vi "Snap_timestamp.vi"(8 "error in":errorcluster, 10 "Camera":T5, 11 "input cluster":T1={"L16 Linear Actuator"="", "XE 1000 Pump"="", "Camera1"="", "Camera2"="", "Img_Capt"=FALSE, "Actuator"=FALSE, "Pump"=FALSE, "Cam 1"=FALSE, "Cam 2"=FALSE, "Empty_Refill"=FALSE, "Crop"=FALSE, "Light intensity"=100, "Exposure Time"=1000.0, "Sample Name"="Test Sample", "Operator"="MRJ", "Calibration 1"=path "C:/Users/au540322/Desktop/IHS_Project/images/Debris/Debris_0/Debris_0_2019_06_01-23-32-49-686.PNG", "Calibration 2"=path "C:/Users/au540322/Desktop/IHS_Project/images/Debris/Debris_0/Debris_0_2019_06_01-23-32-49-686.PNG", "Framerate"=100, "Timeout Sample"=200, "Collection date"="", "Sample size threshold"=500, "Empty start"=1, "Command"="", "Station"="", "Species Name"="", "Other Notes"="", "Aperture"=enum."Item 0", "Image Process Queue Size"=500, "Image Save Queue Size"=500, "Overload threshold"=500, "Max Framerate"=100, "Rectangle 1"={"Left"=0, "Top"=0, "Right"=0, "Bottom"=0, "Rotation"=0.0}, "Rectangle 2"={"Left"=0, "Top"=0, "Right"=0, "Bottom"=0, "Rotation"=0.0}, "Detection Region %"=0.0, "Detect 1"=path "C:/Users/au540322/Desktop/IHS_Project/images/Debris/Debris_0/Debris_0_2019_06_01-23-32-49-686.PNG", "Detect 2"=path "C:/Users/au540322/Desktop/IHS_Project/images/Debris/Debris_0/Debris_0_2019_06_01-23-32-49-686.PNG", "Max large object threshold"=0, "Open(T)/Close(F)"=FALSE, "Img_Capt Begin"=FALSE, "Dispense Speed"=100, "Flush Size"=100, "Location"="Station", "Latitude"="Station", "Longitude"="Station", "Determiner"="Station", "Sex"="Station", "Camera1_Img"=refnum, "Camera2_Img"=refnum, "Img1_Orig_Disp"=refnum, "Img2_Orig_Disp"=refnum, "Img1_Orig_RGB"=refnum, "Img2_Orig_RGB"=refnum, "Blue_Plane_Extract"=refnum, "Subtracted_Plane"=refnum, "Img1_Binary"=refnum, "Img2_Binary"=refnum, "Crop_Mask"=refnum, "Img1_Save"=refnum, "Img2_Save"=refnum, "Img1_Cali_Full"=refnum, "Img2_Cali_Full"=refnum, "Img1_Cali_Detect"=refnum, "Img2_Cali_Detect"=refnum, "Cam 1 queue"=refnum, "Cam 2 queue"=refnum, "Cam 1 - save queue"=refnum, "Cam 2 - save queue"=refnum, "Overlay_Ring"=0, "SystemVersion"=0, "System Serial"="", "Legacy Cam Attributes"=FALSE} {"SystemVersion" items=["Standard", "XL"]; "Overlay_Ring" items=["Session Data", "Extended Setup", "Buffer", "Camera", "Dispenser", "Stats", "Connections"]; "Flush Size" min=1; "Dispense Speed" min=1; "Rectangle 2"."Rotation" format="%.2f"; "Rectangle 2"."Left" scale=0.0..1024.0; "Rectangle 2"."Right" scale=0.0..1024.0; "Rectangle 1"."Rotation" format="%.2f"; "Rectangle 1"."Left" scale=0.0..1024.0; "Rectangle 1"."Right" scale=0.0..1024.0; "Max Framerate" min=1; "Overload threshold" min=1; "Image Save Queue Size" min=1; "Image Process Queue Size" min=1; "Empty start" min=1; "Sample size threshold" min=1; "Framerate" min=1; "Light intensity" scale=0.0..100.0}) -> (0 "error out":errorcluster)   [LabVIEW 2022 SP3]
uses:
  Camera_ID.ctl
  controls/Data.ctl
  <vilib>/userdefined/High Color/IMAQdx.ctl
  <vilib>/vision/Image Controls.llb/IMAQ Image.ctl
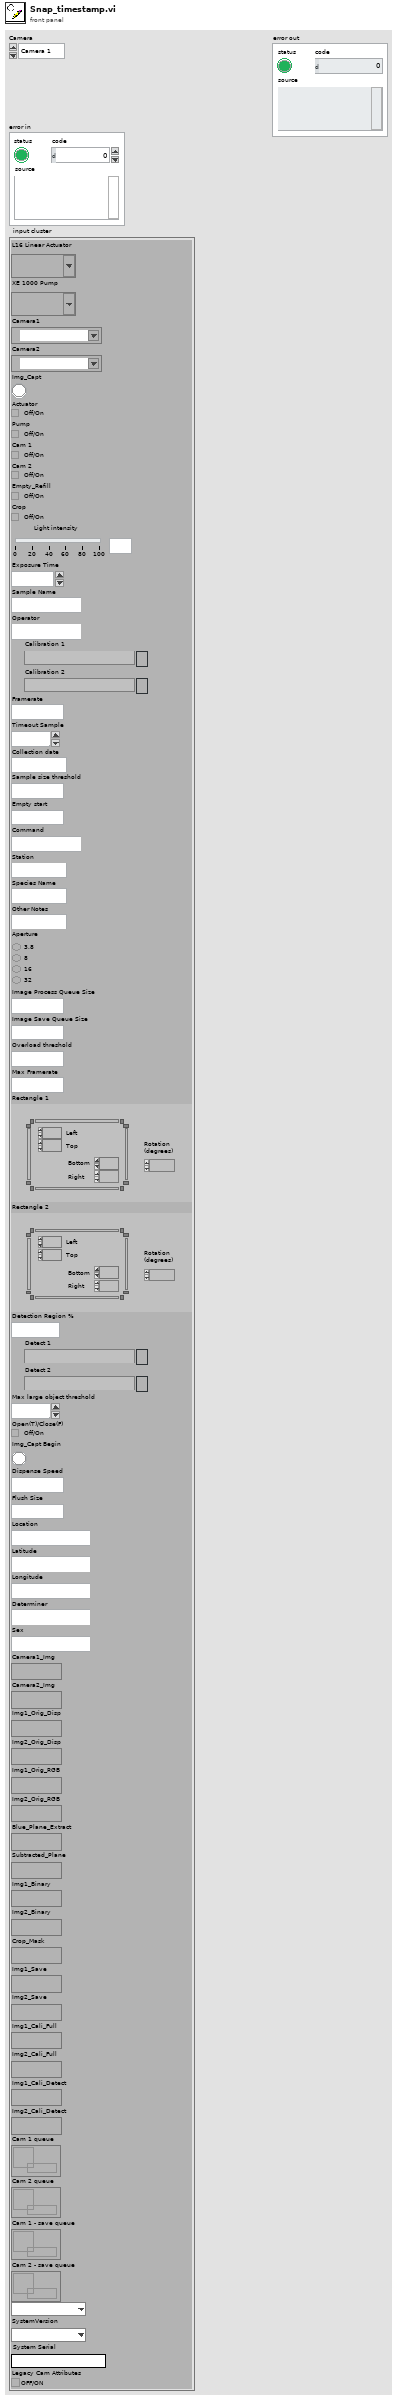
[diagram p1: front panel]
types:
  T1 = typedef "Data.ctl" = cluster{"L16 Linear Actuator":refnum<visa-resource-name>, "XE 1000 Pump":refnum<visa-resource-name>, "Camera1":T2, "Camera2":T2, "Img_Capt":bool, "Actuator":bool, "Pump":bool, "Cam 1":bool, "Cam 2":bool, "Empty_Refill":bool, "Crop":bool, "Light intensity":i32, "Exposure Time":dbl, "Sample Name":string, "Operator":string, "Calibration 1":path, "Calibration 2":path, "Framerate":i32, "Timeout Sample":i32, "Collection date":string, "Sample size threshold":i32, "Empty start":u32, "Command":string, "Station":string, "Species Name":string, "Other Notes":string, "Aperture":enum32{"Item 0", "Item 1", "Item 2", "Item 3"}, "Image Process Queue Size":i32, "Image Save Queue Size":i32, "Overload threshold":i32, "Max Framerate":i32, "Rectangle 1":T3, "Rectangle 2":T3, "Detection Region %":dbl, "Detect 1":path, "Detect 2":path, "Max large object threshold":i32, "Open(T)/Close(F)":bool, "Img_Capt Begin":bool, "Dispense Speed":i32, "Flush Size":i32, "Location":string, "Latitude":string, "Longitude":string, "Determiner":string, "Sex":string, "Camera1_Img":T4, "Camera2_Img":T4, "Img1_Orig_Disp":T4, "Img2_Orig_Disp":T4, "Img1_Orig_RGB":T4, "Img2_Orig_RGB":T4, "Blue_Plane_Extract":T4, "Subtracted_Plane":T4, "Img1_Binary":T4, "Img2_Binary":T4, "Crop_Mask":T4, "Img1_Save":T4, "Img2_Save":T4, "Img1_Cali_Full":T4, "Img2_Cali_Full":T4, "Img1_Cali_Detect":T4, "Img2_Cali_Detect":T4, "Cam 1 queue":refnum<queue>, "Cam 2 queue":refnum<queue>, "Cam 1 - save queue":refnum<queue>, "Cam 2 - save queue":refnum<queue>, "Overlay_Ring":u16, "SystemVersion":u16, "System Serial":string, "Legacy Cam Attributes":bool}
  T2 = typedef "IMAQdx.ctl" = refnum<k21>
  T3 = typedef "IMAQ Rectangle" = cluster{"Left":i32, "Top":i32, "Right":i32, "Bottom":i32, "Rotation":dbl}
  T4 = typedef "IMAQ Image.ctl" = refnum<image>
  T5 = typedef "Camera_ID.ctl" = enum16{"Camera 1", "Camera 2"}
  T6 = cluster{"Timestamp":string, "Image Pixels (U32)":u32[][], "Prev. sample":i32, "Sample Data":dbl[], "output cluster":cluster{"Global Rectangle":i32[], "Contours":cluster{"ID":enum32{"External", "Internal"}, "Type":u32, "Coordinates":i32[]}[]}}
  T7 = cluster{"Global Rectangle":i32[], "Contours":cluster{"ID":enum32{"External", "Internal"}, "Type":u32, "Coordinates":i32[]}[]}
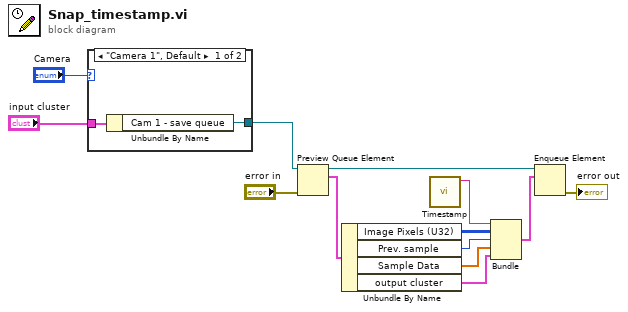
[diagram p0: block diagram]
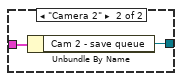
[diagram p2: hidden frame]
diagram:
  n1 = case shown="\"Camera 1\", Default" "Camera" {
    tunnel: [w14 w17] -> w2
    tunnel: "input cluster" -> [w15 w16]
    frame "Camera 1", Default {
      n2 = Unbundle By Name(w15) -> ("Cam 1 - save queue"=w14:refnum<queue>)
    }
    frame "Camera 2" {
      n3 = Unbundle By Name(w16) -> ("Cam 2 - save queue"=w17:refnum<queue>)
    }
  }
  n4 = Preview Queue Element(queue=w2, error in (no error)="error in") -> (queue out=w12:refnum<queue>, element=w11:T6)  [unwired: 1 in, 2 out]
  n5 = Unbundle By Name(w11) -> ("Image Pixels (U32)"=w7:u32[][], "Prev. sample"=w8:i32, "Sample Data"=w9:dbl[], "output cluster"=w10:T7)
  n6 = call "Timestamp.vi"() -> ("Timestamp"=w6:string)  [unwired: 11 in]
  n7 = Bundle("Timestamp"=w6, "Image Pixels (U32)"=w7, "Prev. sample"=w8, "Sample Data"=w9, "output cluster"=w10) -> (w5:T6)  [unwired: 1 in]
  n8 = Enqueue Element(queue=w12, element=w5) -> (error out=→"error out":errorcluster)  [unwired: 2 in, 2 out]
